vi "LVClass_ModalCoef ctor From Legendre Data File.vi"(0 "ModalCoef (const)":refnum<class "ModalCoef.lvclass">, 7 "coefs_file_path":path, 11 "error in (no error)":errorcluster) -> (4 "ModalCoef (new)":refnum<class "ModalCoef.lvclass">, 8 "Comments":string, 15 "error out":errorcluster)   [LabVIEW 2020, in "ModalCoef.lvclass"]
doc: "ModalCoef constructor from modal coefficients file.\n\n<B>ModalCoefIn</B> : Constant Pointer to ModalCoef object.\n<B>ModalCoefOut</B> : Constant Pointer to ModalCoef object.\n<B>type</B> : E_MODAL_T Polynomial basis type.\n<B>coefs_file_path</B> : Modal coefficients file path.\n<B>comments</B> : Comment"
uses:
  ModalCoef.lvclass
  Handle creation.ctl
  WavefrontModalReconstructionType.ctl
  ModalCoef.lvclass/ModalCoef.ctl
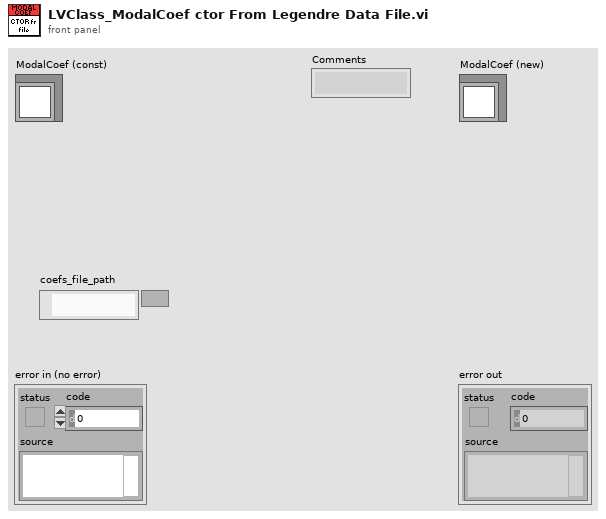
[diagram p1: front panel]
types:
  T1 = typedef "WavefrontModalReconstructionType.ctl" = enum16{"Legendre", "Zernike"}
  T2 = typedef "Handle creation.ctl" = enum16{"By ctor", "By write function"}
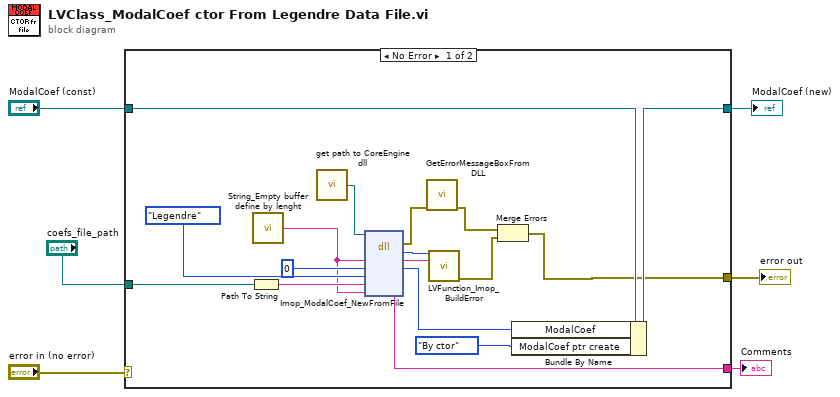
[diagram p0: block diagram]
diagram:
  n1 = case shown="No Error" "error in (no error)" {
    selector: "error in (no error)" -> [_ w25]
    tunnel: [w12 w25] -> w5
    tunnel: [w15 w24] -> w3
    tunnel: "ModalCoef (const)" -> [w16 w24]
    tunnel: "coefs_file_path" -> [w11 _]
    tunnel: [w7 _] -> w1
    frame No Error {
      n2 = Path To String(path=w11) -> (string=w10:string)
      n3 = call "String_Empty buffer define by lenght.vi"() -> ("Empty buffer"=w8:string)  [unwired: 1 in]
      n4 = call "get path to CoreEngine dll.vi"() -> ("path to wavekit library"=w21:path)  [unwired: 14 in, 1 out]
      n5 = dll-call lib="D:/soft/HASO_v3/SVN_trunk/ImOpCoreEngine4_LV2011/DLLs/c_interface_vc100.dll" fn="Imop_ModalCoef_NewFromFile"(path in=w21, "message"=w8, "ModalCoef"=0 ("Pupil"), "TypePhase"=WavefrontModalReconstructionType."Legendre", "coefs_file_path"=w10, "Comments"=w8) -> (error out=w20:errorcluster, "return type"=w22:i32, "message"=w23:string, "ModalCoef"=w18:i64, "Comments"=w7:string)  [unwired: 4 in, 1 out]
      n6 = call "GetErrorMessageBoxFromDLL.vi"("error IN"=w20) -> ("error OUT"=w14:errorcluster)  [unwired: 10 in]
      n7 = call "LVFunction_Imop_BuildError.vi"("code"=w22, "String to Prepend to source (\"\")"=w23) -> ("error out"=w13:errorcluster)  [unwired: 13 in]
      n8 = Merge Errors(w14, w13) -> (w12:errorcluster)
      n9 = Bundle By Name(cluster=w16, "ModalCoef"=w18, "ModalCoef ptr create"=Handle_creation."By ctor" ("Pupil ptr create")) -> (w15:refnum<class "ModalCoef.lvclass">)
    }
    frame Error {
    }
  }
  "error out" <- w5
  "ModalCoef (new)" <- w3
  "Comments" <- w1
